vi "Truncate_cluster_Monitor.vi"(1 "Length":i32=20, 2 "System Monitor Variables":T1={"Time"=[], "LI1CH1"=[], "LI1CH2"=[], "LI2CH1"=[], "LI2CH2"=[], "LI3CH1"=[], "LI3CH2"=[], "Field"=[], "N_Level"=[], "H_Level"=[], "Heat_370"=[], "Sorb_Heat"=[], "Still_Heat"=[], "Capacity"=[], "Loss"=[], "Magnet_Temperature"=[], "Lam_Pressure"=[], "Lam_NValve"=[], "370-T1"=[], "370-T2"=[], "370-T3"=[], "370-T4"=[], "370-T5"=[], "370-R1"=[], "370-R2"=[], "370-R3"=[], "370-R4"=[], "370-R5"=[], "372-T1"=[], "372-T2"=[], "372-T3"=[], "372-T4"=[], "372-T5"=[], "372-T6"=[], "372-R1"=[], "372-R2"=[], "372-R3"=[], "372-R4"=[], "372-R5"=[], "372-R6"=[], "Nada"=[nan], "K2440_Res"=[], "K2440_Current"=[], "VTI_Heater"=[], "VTI_NValve"=[], "LS340_Heater"=[], "K6221_Amplitude"=[], "K6221_Frequency"=[], "Cond_Pressure"=[], "Still_Pressure"=[], "FP_Out_Pressure"=[], "Dump_Pressure"=[], "V1"=[], "V2"=[], "V4"=[], "V5"=[], "V9"=[], "Forepump"=[], "Compressor"=[], "K6221_Offset"=[], "BoxTemp"=[], "By"=[], "Bz"=[], "Phi"=[], "heater-recond (%)"=[], "Dewar Pressure "=[], "JT-SP-Control"=[], "350 T1"=[], "350 T2"=[], "350 T3"=[], "350 T4"=[], "350 R1"=[], "350 R2"=[], "350 R3"=[], "350 R4"=[], "Angle"=[], "VTI CH1"=[], "VTI CH2"=[], "VTI CH3"=[], "ColdTrap"=[], "Mischer Pot"=[], "G1 (mbar)"=[], "G3 (mbar) "=[], "G4 (mbar)"=[], "IVC (mbar)"=[], "P2 (mbar) "=[], "Pot mischer (mbar)"=[], "AVS Control Channel (K)"=[], "AVS Control Channel (RES)"=[], "AVS  Channel 5 (RES) "=[], "LI3CH3"=[], "LI3CH4"=[], "LI1CH3"=[], "LI1CH4"=[], "LI2CH3"=[], "LI2CH4"=[], "Volt"=[], "Watt"=[], "Torque Angle"=[], "Dewar heater (W)"=[], "PSU Voltage"=[], "Turbopump"=[], "372-R7"=[], "372-T7"=[], "SIM921 Ch1"=[], " He3 Temp1"=[], " He3 Temp 2"=[], "LI4CH1"=[], "LI4CH2"=[], "372-T8"=[], "372-R8"=[]}) -> (0 "System Monitor Variables 2":T1={"Time"=[], "LI1CH1"=[], "LI1CH2"=[], "LI2CH1"=[], "LI2CH2"=[], "LI3CH1"=[], "LI3CH2"=[], "Field"=[], "N_Level"=[], "H_Level"=[], "Heat_370"=[], "Sorb_Heat"=[], "Still_Heat"=[], "Capacity"=[], "Loss"=[], "Magnet_Temperature"=[], "Lam_Pressure"=[], "Lam_NValve"=[], "370-T1"=[], "370-T2"=[], "370-T3"=[], "370-T4"=[], "370-T5"=[], "370-R1"=[], "370-R2"=[], "370-R3"=[], "370-R4"=[], "370-R5"=[], "372-T1"=[], "372-T2"=[], "372-T3"=[], "372-T4"=[], "372-T5"=[], "372-T6"=[], "372-R1"=[], "372-R2"=[], "372-R3"=[], "372-R4"=[], "372-R5"=[], "372-R6"=[], "Nada"=[nan], "K2440_Res"=[], "K2440_Current"=[], "VTI_Heater"=[], "VTI_NValve"=[], "LS340_Heater"=[], "K6221_Amplitude"=[], "K6221_Frequency"=[], "Cond_Pressure"=[], "Still_Pressure"=[], "FP_Out_Pressure"=[], "Dump_Pressure"=[], "V1"=[], "V2"=[], "V4"=[], "V5"=[], "V9"=[], "Forepump"=[], "Compressor"=[], "K6221_Offset"=[], "BoxTemp"=[], "By"=[], "Bz"=[], "Phi"=[], "heater-recond (%)"=[], "Dewar Pressure "=[], "JT-SP-Control"=[], "350 T1"=[], "350 T2"=[], "350 T3"=[], "350 T4"=[], "350 R1"=[], "350 R2"=[], "350 R3"=[], "350 R4"=[], "Angle"=[], "VTI CH1"=[], "VTI CH2"=[], "VTI CH3"=[], "ColdTrap"=[], "Mischer Pot"=[], "G1 (mbar)"=[], "G3 (mbar) "=[], "G4 (mbar)"=[], "IVC (mbar)"=[], "P2 (mbar) "=[], "Pot mischer (mbar)"=[], "AVS Control Channel (K)"=[], "AVS Control Channel (RES)"=[], "AVS  Channel 5 (RES) "=[], "LI3CH3"=[], "LI3CH4"=[], "LI1CH3"=[], "LI1CH4"=[], "LI2CH3"=[], "LI2CH4"=[], "Volt"=[], "Watt"=[], "Torque Angle"=[], "Dewar heater (W)"=[], "PSU Voltage"=[], "Turbopump"=[], "372-R7"=[], "372-T7"=[], "SIM921 Ch1"=[], " He3 Temp1"=[], " He3 Temp 2"=[], "LI4CH1"=[], "LI4CH2"=[], "372-T8"=[], "372-R8"=[]})   [LabVIEW 2019]
uses:
  Global/Global Variables/System Monitor Cluster.ctl
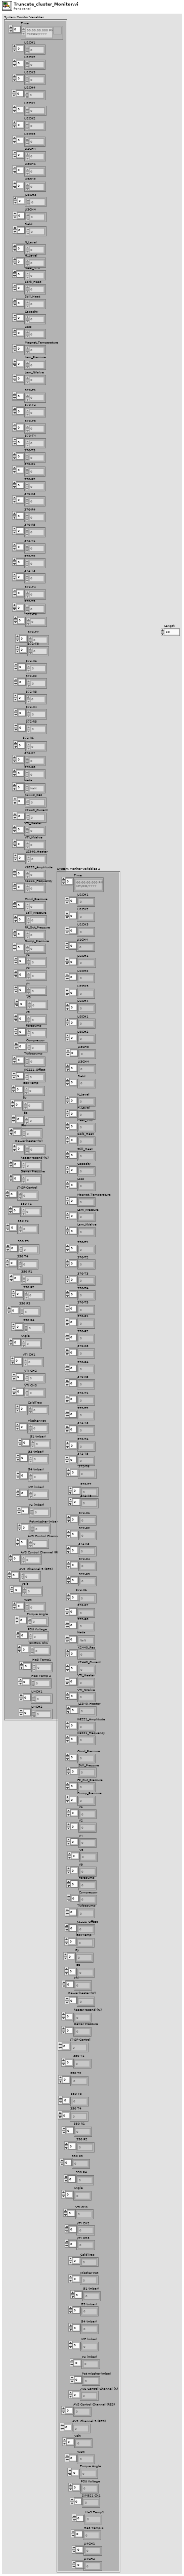
[diagram p1: front panel]
types:
  T1 = typedef "System Monitor Cluster.ctl" = cluster{"Time":timestamp[], "LI1CH1":dbl[], "LI1CH2":dbl[], "LI2CH1":dbl[], "LI2CH2":dbl[], "LI3CH1":dbl[], "LI3CH2":dbl[], "Field":dbl[], "N_Level":dbl[], "H_Level":dbl[], "Heat_370":dbl[], "Sorb_Heat":dbl[], "Still_Heat":dbl[], "Capacity":dbl[], "Loss":dbl[], "Magnet_Temperature":dbl[], "Lam_Pressure":dbl[], "Lam_NValve":dbl[], "370-T1":dbl[], "370-T2":dbl[], "370-T3":dbl[], "370-T4":dbl[], "370-T5":dbl[], "370-R1":dbl[], "370-R2":dbl[], "370-R3":dbl[], "370-R4":dbl[], "370-R5":dbl[], "372-T1":dbl[], "372-T2":dbl[], "372-T3":dbl[], "372-T4":dbl[], "372-T5":dbl[], "372-T6":dbl[], "372-R1":dbl[], "372-R2":dbl[], "372-R3":dbl[], "372-R4":dbl[], "372-R5":dbl[], "372-R6":dbl[], "Nada":dbl[], "K2440_Res":dbl[], "K2440_Current":dbl[], "VTI_Heater":dbl[], "VTI_NValve":dbl[], "LS340_Heater":dbl[], "K6221_Amplitude":dbl[], "K6221_Frequency":dbl[], "Cond_Pressure":dbl[], "Still_Pressure":dbl[], "FP_Out_Pressure":dbl[], "Dump_Pressure":dbl[], "V1":dbl[], "V2":dbl[], "V4":dbl[], "V5":dbl[], "V9":dbl[], "Forepump":dbl[], "Compressor":dbl[], "K6221_Offset":dbl[], "BoxTemp":dbl[], "By":dbl[], "Bz":dbl[], "Phi":dbl[], "heater-recond (%)":dbl[], "Dewar Pressure ":dbl[], "JT-SP-Control":dbl[], "350 T1":dbl[], "350 T2":dbl[], "350 T3":dbl[], "350 T4":dbl[], "350 R1":dbl[], "350 R2":dbl[], "350 R3":dbl[], "350 R4":dbl[], "Angle":dbl[], "VTI CH1":dbl[], "VTI CH2":dbl[], "VTI CH3":dbl[], "ColdTrap":dbl[], "Mischer Pot":dbl[], "G1 (mbar)":dbl[], "G3 (mbar) ":dbl[], "G4 (mbar)":dbl[], "IVC (mbar)":dbl[], "P2 (mbar) ":dbl[], "Pot mischer (mbar)":dbl[], "AVS Control Channel (K)":dbl[], "AVS Control Channel (RES)":dbl[], "AVS  Channel 5 (RES) ":dbl[], "LI3CH3":dbl[], "LI3CH4":dbl[], "LI1CH3":dbl[], "LI1CH4":dbl[], "LI2CH3":dbl[], "LI2CH4":dbl[], "Volt":dbl[], "Watt":dbl[], "Torque Angle":dbl[], "Dewar heater (W)":dbl[], "PSU Voltage":dbl[], "Turbopump":dbl[], "372-R7":dbl[], "372-T7":dbl[], "SIM921 Ch1":dbl[], " He3 Temp1":dbl[], " He3 Temp 2":dbl[], "LI4CH1":dbl[], "LI4CH2":dbl[], "372-T8":dbl[], "372-R8":dbl[]}
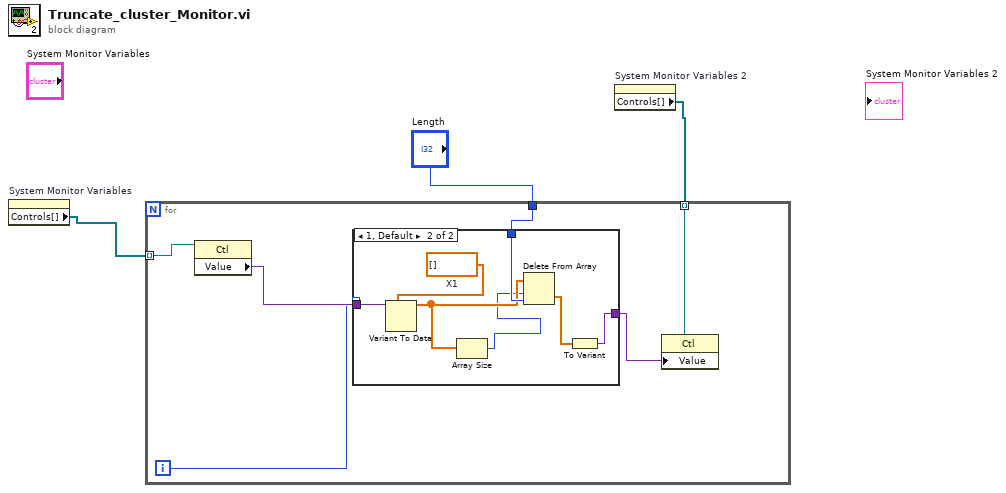
[diagram p0: block diagram]
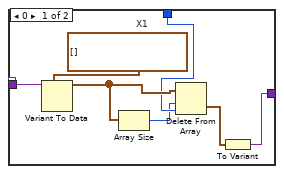
[diagram p2: hidden frame]
diagram:
  n1 = property on="System Monitor Variables" class="Clust (strict)"() -> ("Controls[]"=w2:refnum<vi>[])  [unwired: 2 in, 2 out]
  n2 = property on="System Monitor Variables 2" class="Clust (strict)"() -> ("Controls[]"=w1:refnum<vi>[])  [unwired: 2 in, 2 out]
  n3 = for {
    tunnel: w2 -> [w9] mode=indexing
    tunnel: "Length" -> [w5]
    tunnel: w1 -> [w7] mode=indexing
    i -> [w6]
    n4 = property class="Ctl"(reference=w9) -> ("Value"=w8:variant)  [unwired: 1 in, 2 out]
    n5 = case shown="1, Default" w6 {
      tunnel: w8 -> [w16 w23]
      tunnel: [w14 w21] -> w4
      tunnel: w5 -> [w12 w20]
      frame 0 {
        w15 = timestamp[] []  # X1
        n6 = Variant To Data(type=w15, Variant=w16) -> (data=w13:timestamp[])  [unwired: 1 in, 1 out]
        n7 = Array Size(array=w13) -> (size(s)=w10:i32)
        n8 = Delete From Array(array=w13, length=w10, index=w12) -> (deleted portion=w11:timestamp[])  [unwired: 1 out]
        n9 = To Variant(anything=w11) -> (Variant=w14:variant)
      }
      frame 1, Default {
        w22 = dbl[] []  # X1
        n10 = Variant To Data(type=w22, Variant=w23) -> (data=w19:dbl[])  [unwired: 1 in, 1 out]
        n11 = Array Size(array=w19) -> (size(s)=w17:i32)
        n12 = Delete From Array(array=w19, length=w17, index=w20) -> (deleted portion=w18:dbl[])  [unwired: 1 out]
        n13 = To Variant(anything=w18) -> (Variant=w21:variant)
      }
    }
    n14 = property class="Ctl"(reference=w7, "Value"=w4) -> ()  [unwired: 1 in, 2 out]
  }
